vi "ConfigSource.vi"(6 "Voltage Manual Range (1.0)":dbl=1.0, 7 "Enable Voltage Auto Range (T:Enable)":bool=TRUE, 8 "error in (no error)":errorcluster, 9 "Compliance  Level (0.1)":dbl=0.1, 10 "Voltage Limit (0.0 V)":dbl=1000.0 format="%#_13g", 11 "VISA resource name":refnum<visa-resource-name>) -> (0 "error out":errorcluster, 2 "Output Level (0)":dbl, 3 "VISA resource name out":refnum<visa-resource-name>)   [LabVIEW 2015]
uses:
  Program Files (x86)/National Instruments/LabVIEW 2016/instr.lib/Keithley 24XX/Keithley 24XX.lvlib
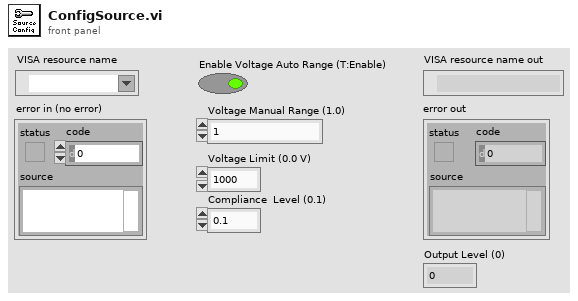
[diagram p1: front panel]
types:
  T1 = cluster{"Baud Rate":u32, "Parity":u16, "Data Bits":u16, "Stop Bits":u16, "Flow Control":u16}
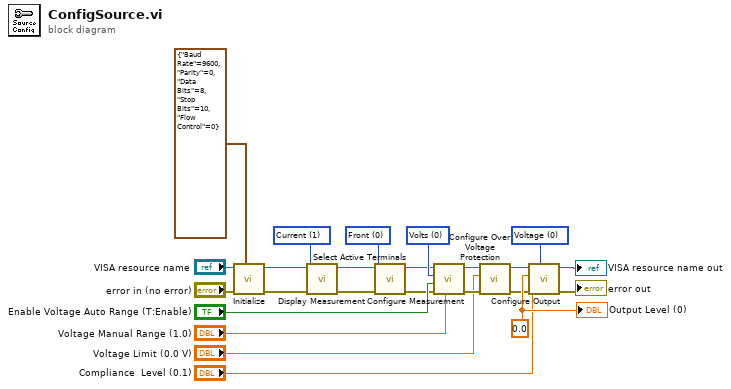
[diagram p0: block diagram]
diagram:
  w1 = u16 1 items=["Voltage", "Current", "Resistance"] ("Displayed Measurement (0: Voltage)")
  w6 = u16 0 items=["Front", "Rear"] ("Active Terminals (0: Front)")
  w18 = 0.0 ("Output Level (0)")
  w19 = u16 0 items=["Voltage", "Current"] ("Source Mode  (0: Voltage)")
  w23 = u16 0 items=["Volts", "Current", "Resistance"] ("Function (0: Volts)")
  n1 = call "Initialize.vi"("Serial Configuration"=T1 {"Baud Rate"=9600, "Parity"=0, "Data Bits"=8, "Stop Bits"=10, "Flow Control"=0}, "error in (no error)"="error in (no error)", "VISA resource name"="VISA resource name") -> ("error out"=w4:errorcluster, "VISA resource name out"=w5:refnum<visa-resource-name>)  [unwired: 7 in]
  n2 = call "Display Measurement.vi"("error in (no error)"=w4, "Displayed Measurement (0: Voltage)"=w1, "VISA resource name"=w5) -> ("error out"=w3:errorcluster, "VISA resource name out"=w2:refnum<visa-resource-name>)  [unwired: 7 in]
  n3 = call "Select Active Terminals.vi"("error in (no error)"=w3, "Active Terminals (0: Front)"=w6, "VISA resource name"=w2) -> ("error out"=w7:errorcluster, "VISA resource name out"=w8:refnum<visa-resource-name>)  [unwired: 7 in]
  n4 = call "Configure Measurement.vi"("Manual Range (1.0)"="Voltage Manual Range (1.0)", "error in (no error)"=w7, "Enable Auto Range (T:Enable)"="Enable Voltage Auto Range (T:Enable)", "Function (0: Volts)"=w23, "VISA resource name"=w8) -> ("error out"=w14:errorcluster, "VISA resource name out"=w15:refnum<visa-resource-name>)  [unwired: 5 in]
  n5 = call "Configure Over Voltage Protection.vi"("error in (no error)"=w14, "Voltage Limit (0.0 V)"="Voltage Limit (0.0 V)", "VISA resource name"=w15) -> ("error out"=w16:errorcluster, "VISA resource name out"=w17:refnum<visa-resource-name>)  [unwired: 7 in]
  n6 = call "Configure Output.vi"("Source Mode  (0: Voltage)"=w19, "error in (no error)"=w16, "Compliance  Level (0.1)"="Compliance  Level (0.1)", "Output Level (0)"=w18, "VISA resource name"=w17) -> ("error out"=→"error out":errorcluster, "VISA resource name out"=→"VISA resource name out":refnum<visa-resource-name>)  [unwired: 5 in]
  "Output Level (0)" <- w18
